vi "Create.vi"(8 "error in (no error)":errorcluster, 9 "TCP":refnum<k5>, 10 "Request":refnum<class "Request.lvclass">) -> (0 "error out":errorcluster, 3 "SSE Client out":refnum<class "SSE Client.lvclass">)   [LabVIEW 2020, in "HTTP Server.lvlib" / "SSE Client.lvclass"]
uses:
  SSE Client.lvclass
  SSE Client.lvclass/SSE Client.ctl
  lv-http-util/HTTP Utils/Request/Request.lvclass
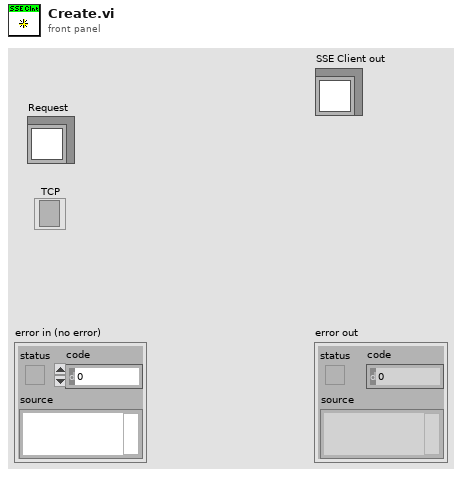
[diagram p1: front panel]
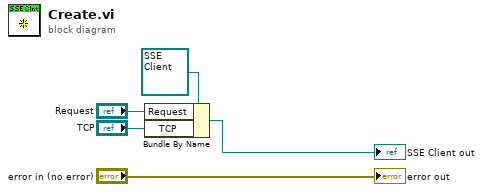
[diagram p0: block diagram]
diagram:
  n1 = Bundle By Name(cluster=refnum<class "SSE Client.lvclass"> refnum ("SSE Client in"), "Request"="Request", "TCP"="TCP") -> (→"SSE Client out":refnum<class "SSE Client.lvclass">)
  "error out" <- "error in (no error)"
